vi "Initialize.vi"(7 "Serial Configuration":cluster{"Baud Rate":u32, "Address":u16}={"Baud Rate"=9600, "Address"=1} {"Address" max=15 step=1; "Baud Rate" items=["300"=300, "600"=600, "1200"=1200, "2400"=2400, "4800"=4800, "9600"=9600, "19200"=19200]}, 8 "error in (no error)":errorcluster, 11 "VISA resource name":refnum<visa-resource-name>) -> (0 "error out":errorcluster, 3 "VISA resource name out":refnum<visa-resource-name>)   [LabVIEW 2021, in "Copy of Kloehn V6 Series.lvlib"]
doc: "Establishes communication with the instrument and places the instrument in a default state needed for other instrument driver operations. Therefore, call this VI before calling other instrument driver VIs for this instrument. Generally, you need to call the Initialize VI only once at the beginning of an application."
uses:
  Copy of Kloehn V6 Series.lvlib
panel:
  # "(c) 2012 National Instruments.  ALL RIGHTS RESERVED."
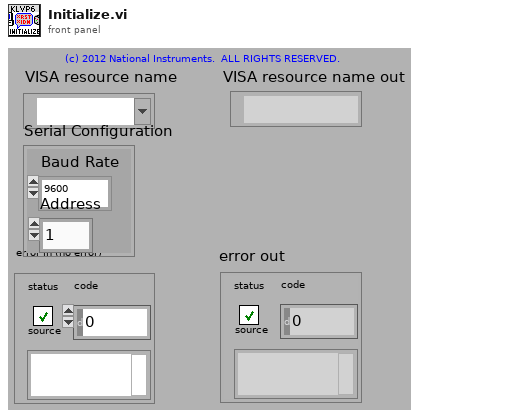
[diagram p1: front panel]
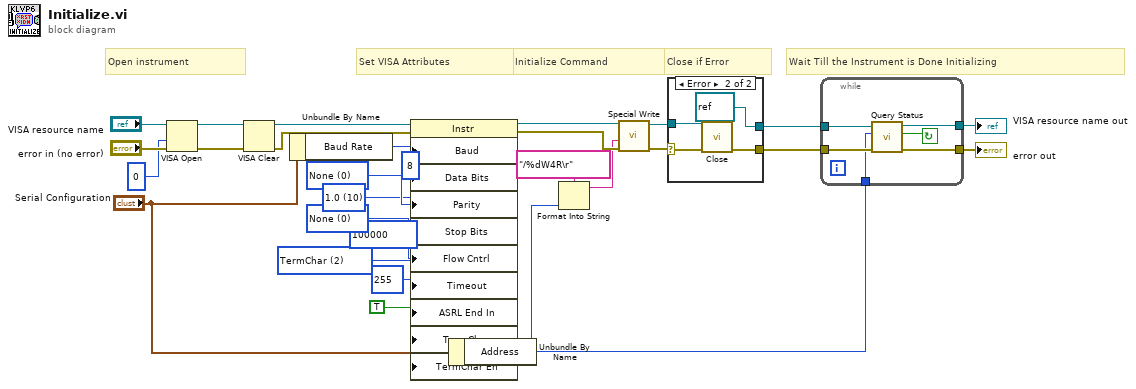
[diagram p0: block diagram]
diagram:
  w12 = u16 2 items=["None", "Last Bit", "TermChar"] ("Serial Settings:End Mode for Reads")
  w14 = u16 0 items=["None", "XON/XOFF", "RTS/CTS", "XON/XOFF & RTS/CTS", "DTR/DSR", "XON/XOFF & DTR/DSR"] ("Serial Settings:Flow Control")
  w15 = u16 10 items=["1.0"=10, "1.5"=15, "2.0"=20] ("Serial Settings:Stop Bits")
  w16 = u16 0 items=["None", "Odd", "Even", "Mark", "Space"] ("Serial Settings:Parity")
  # "Wait Till the Instrument is Done Initializing"
  # "Serial Only"
  # "Set VISA Attributes"
  # "Close if Error"
  # "Send Initialize Command"
  # "Open instrument"
  n1 = VISA Open(access mode=u32 0, error in (no error)="error in (no error)", VISA resource name="VISA resource name") -> (VISA resource name=w21:refnum<visa-resource-name>, error out=w20:errorcluster)  [unwired: 2 in]
  n2 = VISA Clear(VISA resource name=w21, error in (no error)=w20) -> (VISA resource name out=w19:refnum<visa-resource-name>, error out=w18:errorcluster)
  n3 = Unbundle By Name("Serial Configuration") -> ("Baud Rate"=w9:u32)
  n4 = property on="Property Node" class="Instr"(reference=w19, error in=w18, "Baud"=w9, "Data Bits"=u16 8 ("Serial Settings:Data Bits"), "Parity"=w16, "Stop Bits"=w15, "Flow Cntrl"=w14, "Timeout"=u32 100000 ("General Settings:Timeout Value"), "ASRL End In"=w12, "TermChar"=u8 255 ("Message Based Settings:Termination Character"), "TermChar En"=TRUE ("Message Based Settings:Termination Character Enable")) -> (reference out=w23:refnum<visa-resource-name>, error out=w22:errorcluster)
  n5 = Unbundle By Name("Serial Configuration") -> ("Address"=w3:u16)
  n6 = Format Into String(format string="/%dW4R\r" ("Send String"), w3) -> (resulting string=w6:string)  [unwired: 2 in, 1 out]
  n7 = call "Special Write.vi"("error in (no error)"=w22, "Send String"=w6, "VISA resource name"=w23) -> ("error out"=w24:errorcluster, "VISA resource name out"=w25:refnum<visa-resource-name>)  [unwired: 4 in, 3 out]
  n8 = case shown="Error" w24 {
    selector: w24 -> [w29 w33]
    tunnel: [w30 refnum<visa-resource-name> refnum ("VISA resource name out")] -> w5
    tunnel: [w29 w34] -> w4
    tunnel: w25 -> [w30 w31]
    frame No Error {
    }
    frame Error {
      n9 = call "Close.vi"("error in (no error)"=w33, "VISA resource name"=w31) -> ("error out"=w34:errorcluster)  [unwired: 9 in]
    }
  }
  n10 = while {
    tunnel: w5 -> [w40]
    tunnel: w4 -> [w39]
    tunnel: w3 -> [w38]
    tunnel: [w37] -> w2
    tunnel: [w36] -> w1
    stop <- w35 continue-if-true
    n11 = call "Query Status.vi"("error in (no error)"=w39, "Address (1)"=w38, "VISA resource name"=w40) -> ("error out"=w36:errorcluster, "Status"=w35:bool, "VISA resource name out"=w37:refnum<visa-resource-name>)  [unwired: 6 in]
  }
  "VISA resource name out" <- w2
  "error out" <- w1
